vi "Stop Client.vi"   [LabVIEW 2011]
panel:
  # "Please Wait"
types:
  T1 = enum16{"Standard", "Buffered", "CRLF", "Immediate"}
  T2 = enum32{"invalid app kind", "Development System", "Run Time System", "Student Edition", "Embedded LabVIEW", "Evaluation", "Custom"}
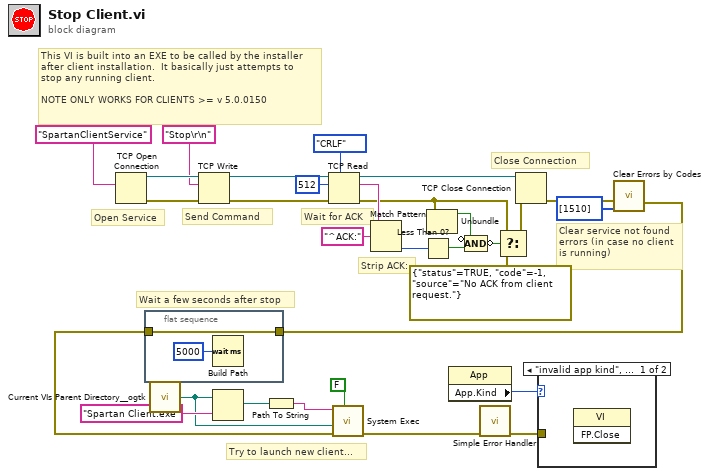
[diagram p0: block diagram]
diagram:
  # "Wait a few seconds after stop"
  # "Try to launch new client..."
  # "Clear service not found\nerrors (in case no client\nis running)"
  # "This VI is built into an EXE to be called by the installer\nafter client installation.  It basically just attempts to\nstop any running client. \n\nNOTE ONLY WORKS FOR CLIENTS >= v 5.0.0150"
  # "Strip ACK:"
  # "Close Connection"
  # "Wait for ACK"
  # "Send Command"
  # "Open Service"
  n1 = TCP Open Connection(remote port or service name="SpartanClientService") -> (connection ID=w29:refnum<k5>, error out=w28:errorcluster)  [unwired: 1 in, 3 out]
  n2 = flat-sequence {
    tunnel: w2 -> [w31]
    tunnel: [w31] -> w1
    frame #0 {
      n3 = Wait (ms)(milliseconds to wait=u32 5000) -> ()  [unwired: 1 out]
    }
  }
  n4 = call "Current VIs Parent Directory__ogtk.vi"() -> ("Parent Directory (+ Relative)"=w5:path)  [unwired: 5 out]
  n5 = TCP Write(connection ID=w29, data in="Stop\r\n" ("regular expression"), error in (no error)=w28) -> (connection ID out=w27:refnum<k5>, error out=w26:errorcluster)  [unwired: 2 out]
  n6 = Build Path(base path=w5, name or relative path="Spartan Client.exe") -> (appended path=w4:path)
  n7 = Path To String(path=w4) -> (string=w3:string)
  n8 = TCP Read(connection ID=w27, bytes to read=512, error in (no error)=w26, 7:T1."CRLF" ("mode (standard)")) -> (connection ID out=w22:refnum<k5>, data out=w23:string, error out=w16:errorcluster)  [unwired: 1 out]
  n9 = call <vilib>:"System Exec.vi"("wait until completion? (T)"=FALSE, "error in (no error)"=w1, "working directory"=w5, "command line"=w3) -> ("error out"=w6:errorcluster)  [unwired: 2 in, 5 out]
  n10 = Match Pattern(string=w23, regular expression="^ACK:") -> (offset past match=w20:i32)  [unwired: 4 out]
  n11 = Less Than 0?(x=w20) -> (x < 0?=w18:bool)
  n12 = Unbundle(w16) -> ("status"=w17:bool)  [unwired: 2 out]
  n13 = property class="App"() -> ("App.Kind"=w11:T2)  [unwired: 2 in, 2 out]
  n14 = Compound Arithmetic op=AND(invert w17, w18) -> (invert w19:bool)
  n15 = call <vilib>:"Simple Error Handler.vi"("error in (no error)"=w6) -> ("error out"=w12:errorcluster)  [unwired: 1 in, 7 out]
  n16 = Select(t=w16, s=w19, f=errorcluster {"status"=TRUE, "code"=-1, "source"="No ACK from client request."} ("t")) -> (s? t:f=w15:errorcluster)
  n17 = TCP Close Connection(connection ID=w22, error in (no error)=w15) -> (error out=w10:errorcluster)  [unwired: 2 out]
  n18 = case shown="\"invalid app kind\", Default" w11 {
    tunnel: w12 -> [_ _]
    frame "invalid app kind", Default {
      n19 = invoke class="VI" method="FP.Close"() -> ()  [unwired: 3 in, 3 out]
    }
    frame "Development System" {
    }
  }
  n20 = call "Clear Errors by Codes.vi"("Error Codes\nto Clear (Empty)"=i32[] [1510] ("Error Codes\nto Clear (Empty)"), "error in (no error)"=w10) -> ("error out"=w2:errorcluster)  [unwired: 5 out]
